vi "USBClient2Sub.vi"() -> ()   [LabVIEW 2018]
uses:
  <vilib>/daq.io/MQTT LabVIEW Client/Controls/Connect_Flags.ctl
  <vilib>/daq.io/MQTT LabVIEW Client/Controls/QoS.ctl
  <vilib>/daq.io/MQTT LabVIEW Client/Controls/DUP_Flag.ctl
  <vilib>/daq.io/MQTT LabVIEW Client/Controls/Retain_Flag.ctl
  <vilib>/DAQmx/write.llb/DAQmx Write (Analog DBL 1Chan 1Samp).vi
  <vilib>/DAQmx/create/channels.llb/DAQmx Create Channel (AO-Voltage-Basic).vi
  <vilib>/DAQmx/miscellaneous.llb/DAQmx Fill In Error Info.vi
  <vilib>/daq.io/MQTT LabVIEW Client/MQTT_Functions.lvlib
panel:
  in  "stop":bool
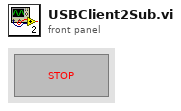
[diagram p1: front panel]
types:
  T1 = typedef "MQTT_Functions.lvlib/QoS.ctl" = enum8{"At most once", "At least once", "Exactly once", "Reserved"}
  T2 = typedef "MQTT_Functions.lvlib/DUP_Flag.ctl" = bool
  T3 = typedef "MQTT_Functions.lvlib/Retain_Flag.ctl" = bool
  T4 = cluster{"QoS":T1, "DUP":T2, "Retain":T3, "Keep Alive (sec)":u16}
  T5 = typedef "MQTT_Functions.lvlib/Connect_Flags.ctl" = cluster{"user name":bool, "password":bool, "will retain":bool, "will flag":bool, "clean session":bool, "reserved":bool, "will QoS":T1}
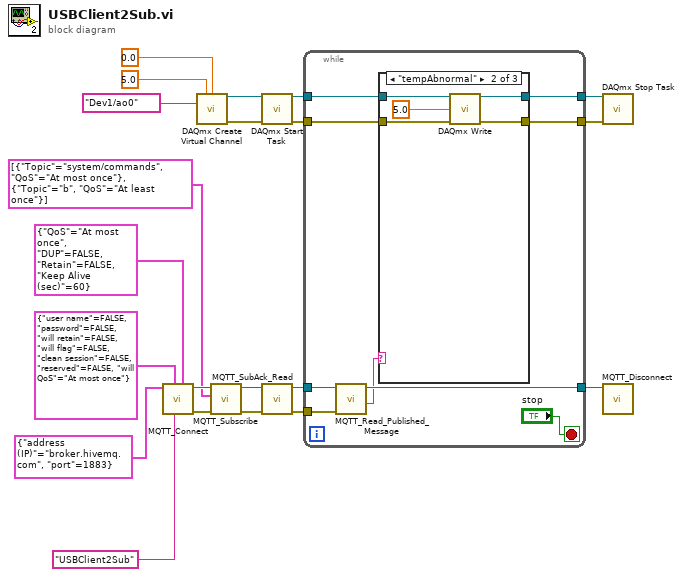
[diagram p0: block diagram]
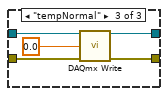
[diagram p3: hidden frame]
diagram:
  n1 = call <vilib>:"MQTT_Connect.vi"("Connect Meta"=T4 {"QoS"=enum."At most once", "DUP"=FALSE, "Retain"=FALSE, "Keep Alive (sec)"=60}, "Client ID"="USBClient2Sub", "Connect Flags"=T5 {"user name"=FALSE, "password"=FALSE, "will retain"=FALSE, "will flag"=FALSE, "clean session"=FALSE, "reserved"=FALSE, "will QoS"=enum."At most once"}, "MQTT Broker"=cluster{"address (IP)":string, "port":u16} {"address (IP)"="broker.hivemq.com", "port"=1883}) -> ("error out"=w17:errorcluster, "connection ID out"=w16:refnum<k5>)  [unwired: 5 in, 1 out]
  n2 = call-poly <vilib>:"DAQmx Create Virtual Channel.vi"("maximum value"=5.0, "minimum value"=0.0, "physical channels"=tag "Dev1/ao0") -> ("task out"=w9:refnum<k21>, "error out"=w8:errorcluster)  [unwired: 11 in]
  n3 = call <vilib>:"MQTT_Subscribe.vi"("error in (no error)"=w17, "Subscription Info Array"=cluster{"Topic":string, "QoS":T1}[] [{"Topic"="system/commands", "QoS"=enum."At most once"}, {"Topic"="b", "QoS"=enum."At least once"}], "connection ID"=w16) -> ("error out"=w14:errorcluster, "connection ID out"=w13:refnum<k5>)  [unwired: 7 in]
  n4 = call <vilib>:"DAQmx Start Task.vi"("task/channels in"=w9, "error in"=w8) -> ("task out"=w7:refnum<k21>, "error out"=w6:errorcluster)  [unwired: 12 in]
  n5 = call <vilib>:"MQTT_SubAck_Read.vi"("error in (no error)"=w14, "connection ID"=w13) -> ("error out"=w11:errorcluster, "connection ID out"=w12:refnum<k5>)  [unwired: 7 in, 1 out]
  n6 = while {
    tunnel: w12 -> [w29]
    tunnel: w11 -> [w30]
    tunnel: [w27] -> w10
    tunnel: w7 -> [w25]
    tunnel: w6 -> [w24]
    tunnel: [w23] -> w2
    tunnel: [w22] -> w1
    stop <- "stop" stop-if-true
    n7 = call <vilib>:"MQTT_Read_Published_Message.vi"("error in (no error)"=w30, "connection ID"=w29) -> ("Message"=w26:string, "connection ID out"=w27:refnum<k5>)  [unwired: 4 in, 4 out]
    n8 = case shown="\"tempAbnormal\"" w26 {
      tunnel: w25 -> [w32 w37 w42]
      tunnel: w24 -> [w31 w36 w41]
      tunnel: [w32 w34 w39] -> w23
      tunnel: [w31 w33 w38] -> w22
      frame "False", Default {
      }
      frame "tempAbnormal" {
        n9 = call-poly <vilib>:"DAQmx Write.vi"("task/channels in"=w37, "data"=5.0, "error in"=w36) -> ("task out"=w34:refnum<k21>, "error out"=w33:errorcluster)  [unwired: 10 in, 1 out]
      }
      frame "tempNormal" {
        n10 = call-poly <vilib>:"DAQmx Write.vi"("task/channels in"=w42, "data"=0.0, "error in"=w41) -> ("task out"=w39:refnum<k21>, "error out"=w38:errorcluster)  [unwired: 10 in, 1 out]
      }
    }
  }
  n11 = call <vilib>:"DAQmx Stop Task.vi"("task/channels in"=w2, "error in"=w1) -> ()  [unwired: 12 in, 2 out]
  n12 = call <vilib>:"MQTT_Disconnect.vi"("connection ID"=w10) -> ()  [unwired: 10 in, 1 out]
